vi "对称性.vi"(9 "索引":i32, 10 "定点":dbl, 11 "XY图":cluster{dbl[], dbl[]}[](graph)) -> (3 "对称性":dbl)   [LabVIEW 2020]
uses:
  <vilib>/Analysis/NI_AAL_Geometry.lvlib
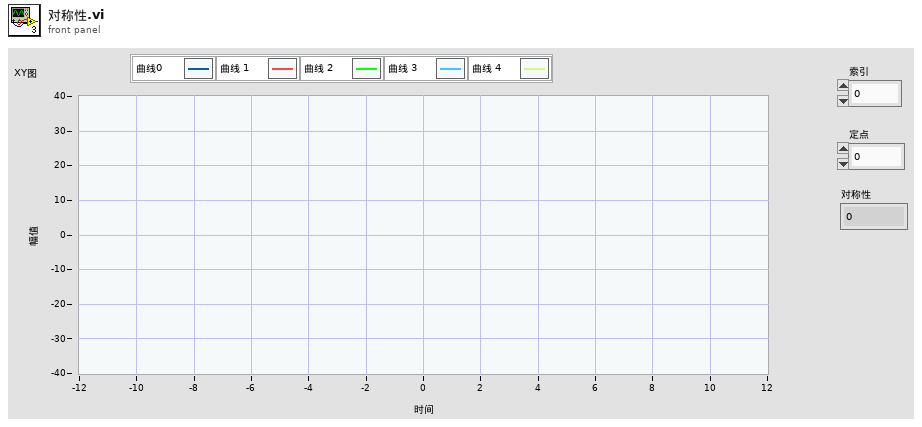
[diagram p1: front panel]
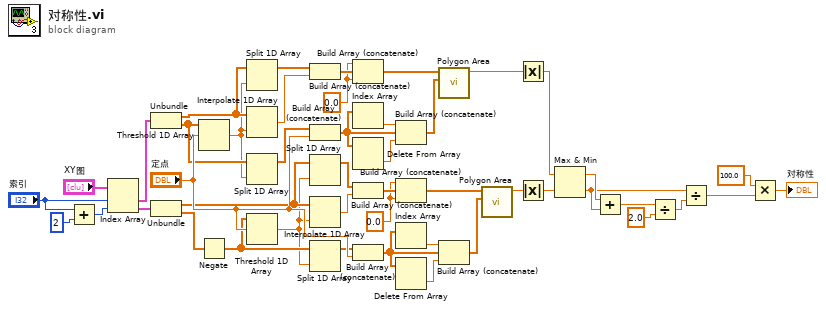
[diagram p0: block diagram]
diagram:
  w28 = 0.0
  w27 = 0.0
  n1 = Add(x="索引", y=2) -> (x+y=w16:i32)
  n2 = Index Array(array="XY图", index #1="索引", index #2=w16) -> (element #1=w32:cluster{dbl[], dbl[]}, element #2=w18:cluster{dbl[], dbl[]})
  n3 = Unbundle(w32) -> (w29:dbl[], w31:dbl[])
  n4 = Unbundle(w18) -> (w10:dbl[], w30:dbl[])
  n5 = Threshold 1D Array(2:"定点", 3:w31) -> (0:w4:dbl)  [unwired: 1 in]
  n6 = Negate(x=w30) -> (-x=w9:dbl[])
  n7 = Split 1D Array(array=w29, index=w4) -> (first subarray=w8:dbl[])  [unwired: 1 out]
  n8 = Interpolate 1D Array(1:w4, 2:w29) -> (0:w3:dbl)
  n9 = Split 1D Array(array=w31, index=w4) -> (first subarray=w7:dbl[])  [unwired: 1 out]
  n10 = Threshold 1D Array(2:"定点", 3:w9) -> (0:w2:dbl)  [unwired: 1 in]
  n11 = Build Array (concatenate)(w8, w3) -> (w35:dbl[])
  n12 = Build Array (concatenate)(w7, "定点") -> (w37:dbl[])
  n13 = Split 1D Array(array=w10, index=w2) -> (first subarray=w5:dbl[])  [unwired: 1 out]
  n14 = Interpolate 1D Array(1:w2, 2:w10) -> (0:w1:dbl)
  n15 = Split 1D Array(array=w9, index=w2) -> (first subarray=w6:dbl[])  [unwired: 1 out]
  n16 = Build Array (concatenate)(w27, w35, w27) -> (w14:dbl[])
  n17 = Index Array(array=w37) -> (element=w36:dbl)  [unwired: 1 in]
  n18 = Delete From Array(array=w37) -> (deleted portion=w38:dbl)  [unwired: 2 in, 1 out]
  n19 = Build Array (concatenate)(w5, w1) -> (w42:dbl[])
  n20 = Build Array (concatenate)(w6, "定点") -> (w41:dbl[])
  n21 = Build Array (concatenate)(w36, w37, w38) -> (w13:dbl[])
  n22 = Build Array (concatenate)(w28, w42, w28) -> (w12:dbl[])
  n23 = Index Array(array=w41) -> (element=w40:dbl)  [unwired: 1 in]
  n24 = Delete From Array(array=w41) -> (deleted portion=w39:dbl)  [unwired: 2 in, 1 out]
  n25 = call <vilib>:"Polygon Area.vi"("Y"=w13, "X"=w14) -> ("signed area"=w34:dbl)  [unwired: 8 in, 1 out]
  n26 = Build Array (concatenate)(w40, w41, w39) -> (w11:dbl[])
  n27 = call <vilib>:"Polygon Area.vi"("Y"=w11, "X"=w12) -> ("signed area"=w33:dbl)  [unwired: 8 in, 1 out]
  n28 = Absolute Value(x=w34) -> (abs(x)=w26:dbl)
  n29 = Absolute Value(x=w33) -> (abs(x)=w25:dbl)
  n30 = Max & Min(x=w26, y=w25) -> (max(x,y)=w24:dbl, min(x,y)=w21:dbl)
  n31 = Add(x=w24, y=w21) -> (x+y=w23:dbl)
  n32 = Divide(x=w23, y=2.0) -> (x/y=w20:dbl)
  n33 = Divide(x=w21, y=w20) -> (x/y=w19:dbl)
  n34 = Multiply(x=100.0, y=w19) -> (x*y=→"对称性":dbl)
